vi "PV ActiveLine - FormatMode.vi"(7 "W/R":bool, 8 "Fehler (Eingang)":errorcluster, 9 "Number Format":i8(ring) items=["X.X", "X.XESY"], 11 "Referenz in":refnum<visa-resource-name>) -> (0 "Cluster (Ausgang)":errorcluster, 1 "Read Status":u16(ring) items=["Read Failed", "Read Ok"], 2 "Number Format Out":i8(ring) items=["X.X", "X.XESY"], 3 "Referenz out":refnum<visa-resource-name>)   [LabVIEW 2013, in "PV ActiveLine.lvlib"]
doc: "FMT - Number Format\n\nTransmit: FMT [,a]\nReceive: a\n\nNumber format (measurement value),\na =\n0 –> Floating point format, if possible (default)\n1 –> Exponential format"
uses:
  <instrlib>/PV ActiveLine/PV ActiveLine.lvlib
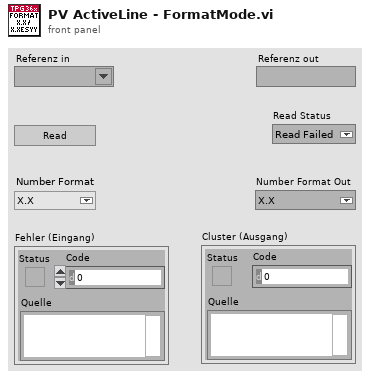
[diagram p1: front panel]
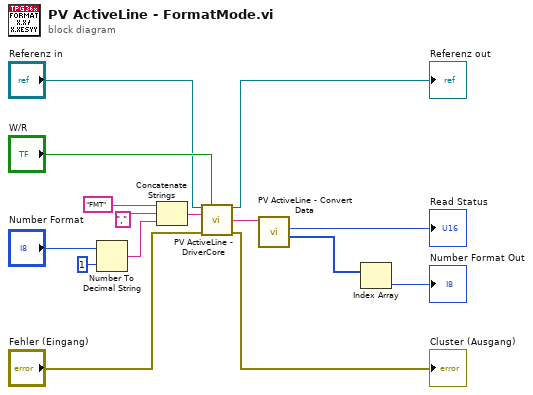
[diagram p0: block diagram]
diagram:
  n1 = Number To Decimal String(number="Number Format", width (-)=i16 1) -> (decimal integer string=w12:string)
  n2 = Concatenate Strings("FMT" ("Command"), "," ("Command"), w12) -> (w9:string)
  n3 = call <instrlib>:"PV ActiveLine - DriverCore.vi"("Referenz in"="Referenz in", "Write/Read"="W/R", "Command"=w9, "Fehler (Eingang)"="Fehler (Eingang)") -> ("Referenz out"=→"Referenz out":refnum<visa-resource-name>, "String Out"=w4:string, "Cluster (Ausgang)"=→"Cluster (Ausgang)":errorcluster)  [unwired: 9 in]
  n4 = call <instrlib>:"PV ActiveLine - Convert Data.vi"("String in"=w4) -> ("Integer Out"=w3:i32[], "Read Status"=→"Read Status":u16)  [unwired: 7 in, 2 out]
  n5 = Index Array(array=w3) -> (element=→"Number Format Out":i32)  [unwired: 1 in]
